vi "Send Result Data Update the Self.vi"(7 "Message Priority (Normal)":T2=enum."Normal", 8 "error in (no error)":errorcluster, 10 "Report Data":T1={"Schema"="", "Test Socket"="", "Start Test Cycle"="", "Stop Test Cycle"="", "Test Mode"="", "Frame Type"="fe_frame_log"}, 11 "Message Enqueuer":refnum<class "Message Enqueuer.lvclass">) -> (0 "error out":errorcluster, 3 "Message Enqueuer out":refnum<class "Message Enqueuer.lvclass">)   [LabVIEW 2023, in "Data Analysis.lvlib" / "Import Export SQL.lvlib" / "Result Data Update the Self Msg.lvclass"]
doc: "This VI sends the message to an actor."
uses:
  Result Data Update the Self Msg.lvclass
  Result Data Update the Self Msg.lvclass/Result Data Update the Self Msg.ctl
  <vilib>/ActorFramework/Message Enqueuer/Message Enqueuer.lvclass
  C:/Program Files/National Instruments/LabVIEW 2023/vi.lib/ActorFramework/Message/Message.lvclass
  D:/eDCU LTT/VT LTT Project/Source Code/Data Analysis/Import Export SQL/Import Export Messages/Result Data Update the Self Msg/Result Data Update the Self Msg.lvclass
  <vilib>/ActorFramework/Message Enqueuer/Message Priority.ctl
  Control/Report.ctl
  Data Analysis.lvlib
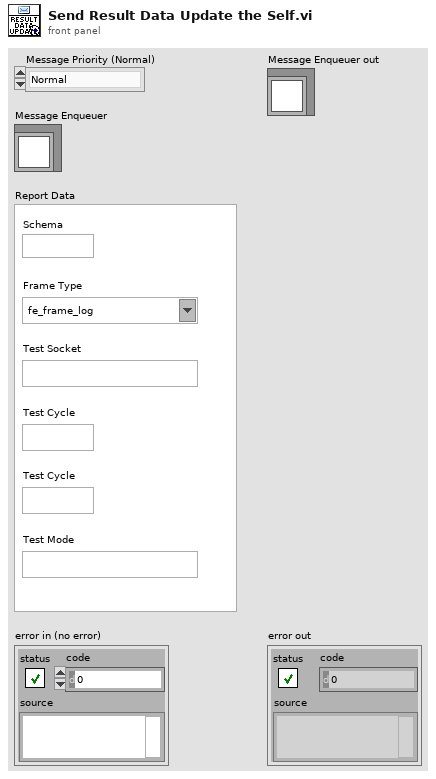
[diagram p1: front panel]
types:
  T1 = typedef "Data Analysis.lvlib/Report.ctl" = cluster{"Schema":string, "Test Socket":string, "Start Test Cycle":string, "Stop Test Cycle":string, "Test Mode":string, "Frame Type":string}
  T2 = typedef "Actor Framework.lvlib/Message Enqueuer.lvclass/Message Priority.ctl" = enum16{"Low", "Normal", "High"}
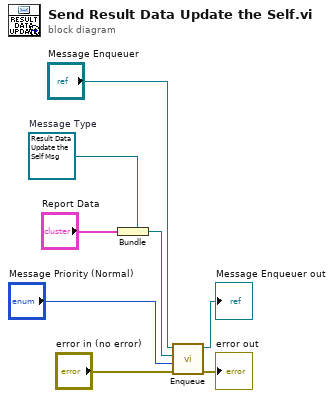
[diagram p0: block diagram]
diagram:
  w5 = refnum<class "Result Data Update the Self Msg.lvclass"> refnum  # Message Type
  n1 = Bundle(cluster=w5, "Report Data") -> (w4:refnum<class "Result Data Update the Self Msg.lvclass">)
  n2 = call <vilib>:"Enqueue.vi"("error in (no error)"="error in (no error)", "Message Priority (Normal)"="Message Priority (Normal)", "Message"=w4, "Message Enqueuer in"="Message Enqueuer") -> ("error out"=→"error out":errorcluster, "Message Enqueuer in"=→"Message Enqueuer out":refnum<class "Message Enqueuer.lvclass">)  [unwired: 6 in]
